vi "FileRichInfo2String.vi"   [LabVIEW 2015]
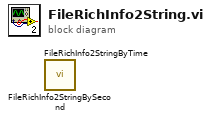
[diagram p0: block diagram]
diagram:
  n1 = call "FileRichInfo2StringBySecond.vi"() -> ()  [unwired: 9 in, 1 out]
  n2 = call "FileRichInfo2StringByTime.vi"() -> ()  [unwired: 9 in, 1 out]
